vi "calcLoopCheckTimes.vi"(8 "error in (no error)":errorcluster, 11 "LoopTimer in":refnum<class "LoopTimer.lvclass">) -> (0 "error out":errorcluster, 3 "LoopTimer out":refnum<class "LoopTimer.lvclass">)   [LabVIEW 2013, in "ComponentData.lvlib" / "LoopTimer.lvclass"]
uses:
  <userlib>/Common/Component/common_application/RT/ComponentData/LoopTimer/LoopTimer.lvclass
  <userlib>/Common/Component/common_application/RT/ComponentData/LoopTimer/LoopTimer.lvclass/LoopTimer.ctl
  <userlib>/Common/Component/common_application/RT/ComponentData/ConfigurationHandler/LoopConfig/LoopConfig.lvclass
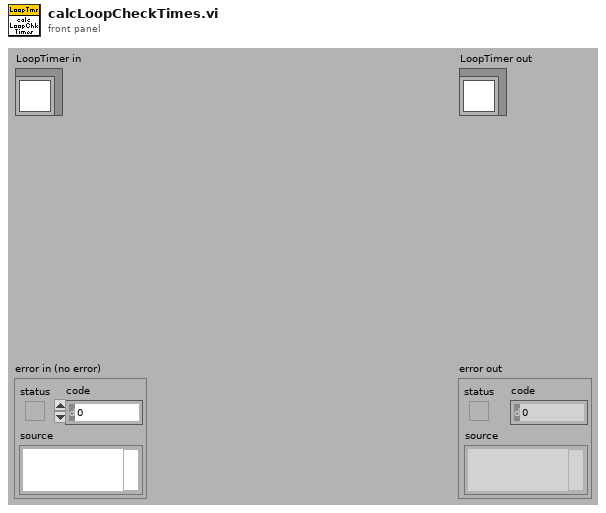
[diagram p1: front panel]
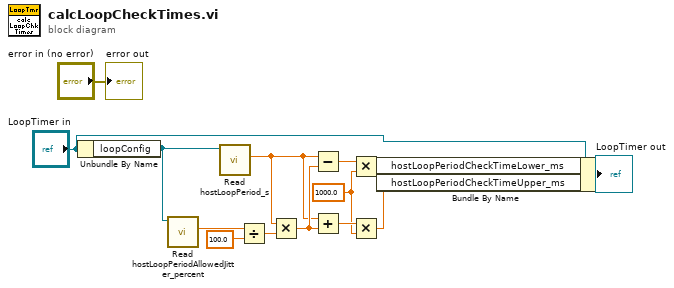
[diagram p0: block diagram]
diagram:
  w6 = 1000.0 ("y")
  n1 = Unbundle By Name("LoopTimer in") -> ("loopConfig"=w11:refnum<class "LoopConfig.lvclass">)
  n2 = call <userlib>:"Read hostLoopPeriodAllowedJitter_percent.vi"("LoopConfig in"=w11) -> ("hostLoopPeriodAllowedJitter_percent"=w3:dbl)  [unwired: 8 in, 2 out]
  n3 = call <userlib>:"Read hostLoopPeriod_s.vi"("LoopConfig in"=w11) -> ("hostLoopPeriod_s"=w4:dbl)  [unwired: 8 in, 2 out]
  n4 = Divide(x=w3, y=100.0) -> (x/y=w9:dbl)
  n5 = Multiply(x=w4, y=w9) -> (x*y=w7:dbl)
  n6 = Subtract(x=w4, y=w7) -> (x-y=w5:dbl)
  n7 = Add(x=w4, y=w7) -> (x+y=w8:dbl)
  n8 = Multiply(x=w5, y=w6) -> (x*y=w2:dbl)
  n9 = Multiply(x=w8, y=w6) -> (x*y=w1:dbl)
  n10 = Bundle By Name(cluster="LoopTimer in", "hostLoopPeriodCheckTimeLower_ms"=w2, "hostLoopPeriodCheckTimeUpper_ms"=w1) -> (→"LoopTimer out":refnum<class "LoopTimer.lvclass">)
  "error out" <- "error in (no error)"
